vi "Data.Engine.DynamicConfigInitialize.vi"(8 "error in":errorcluster, 10 "Data Access info":T3 {"Read"."Refs"."Data Reference" format="%.0x"; "Write"."Refs"."Data Reference" format="%.0x"; "ReadWrite"."Refs" format="%.0x"}, 11 "Data Access Engine":refnum<class "Data Access Engine.lvclass">) -> (0 "error out":errorcluster, 3 "Data Access Engine":refnum<class "Data Access Engine.lvclass">)   [LabVIEW 2023, in "Data Access Engine.lvlib" / "Data Access Engine.lvclass"]
uses:
  Data Access Engine.lvclass
  Data Access Engine.lvclass/Data Access Engine.ctl
  Access Type Classes/Read/Read.lvclass
  Access Type Classes/Write/Write.lvclass
  Access Type Classes/ReadWrite/ReadWrite.lvclass
  <vilib>/NI VeriStand/Custom Device API/Data Reference.ctl
  <vilib>/NI VeriStand/Custom Device API/Custom Device API.lvlib
  <vilib>/NI VeriStand/Custom Device API/Block Data Reference.ctl
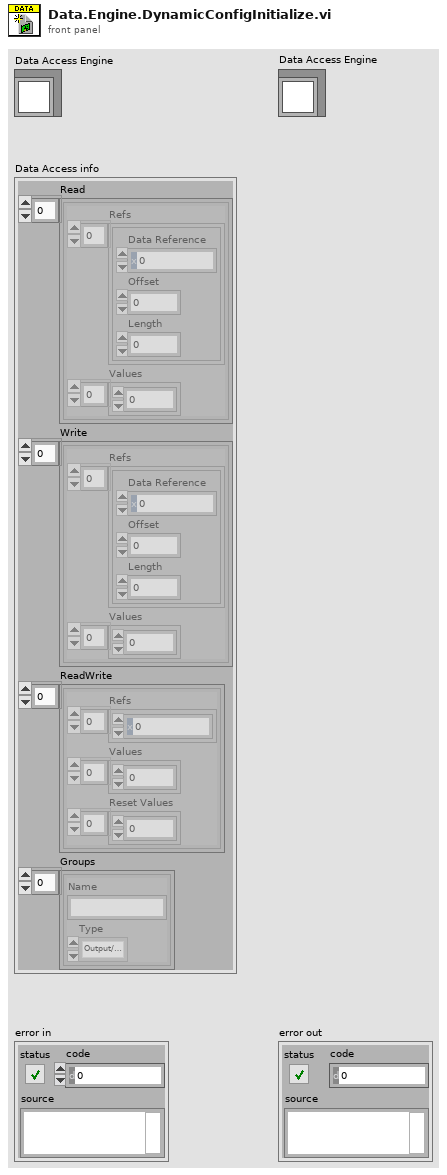
[diagram p1: front panel]
types:
  T1 = typedef "Custom Device API.lvlib/Block Data Reference.ctl" = cluster{"Data Reference":T2, "Offset":u64, "Length":u64}
  T2 = typedef "Custom Device API.lvlib/Data Reference.ctl" = i32
  T3 = cluster{"Read":cluster{"Refs":T1[], "Values":dbl[]}[], "Write":cluster{"Refs":T1[], "Values":dbl[]}[], "ReadWrite":cluster{"Refs":T2[], "Values":dbl[], "Reset Values":dbl[]}[], "Groups":cluster{"Name":string, "Type":enum16{"Output/Write", "Input/Read", "Input/ReadWrite"}}[]}
  T4 = cluster{"Name":string, "Type":enum16{"Output/Write", "Input/Read", "Input/ReadWrite"}}[]
  T5 = cluster{"Refs":T2[], "Values":dbl[], "Reset Values":dbl[]}[]
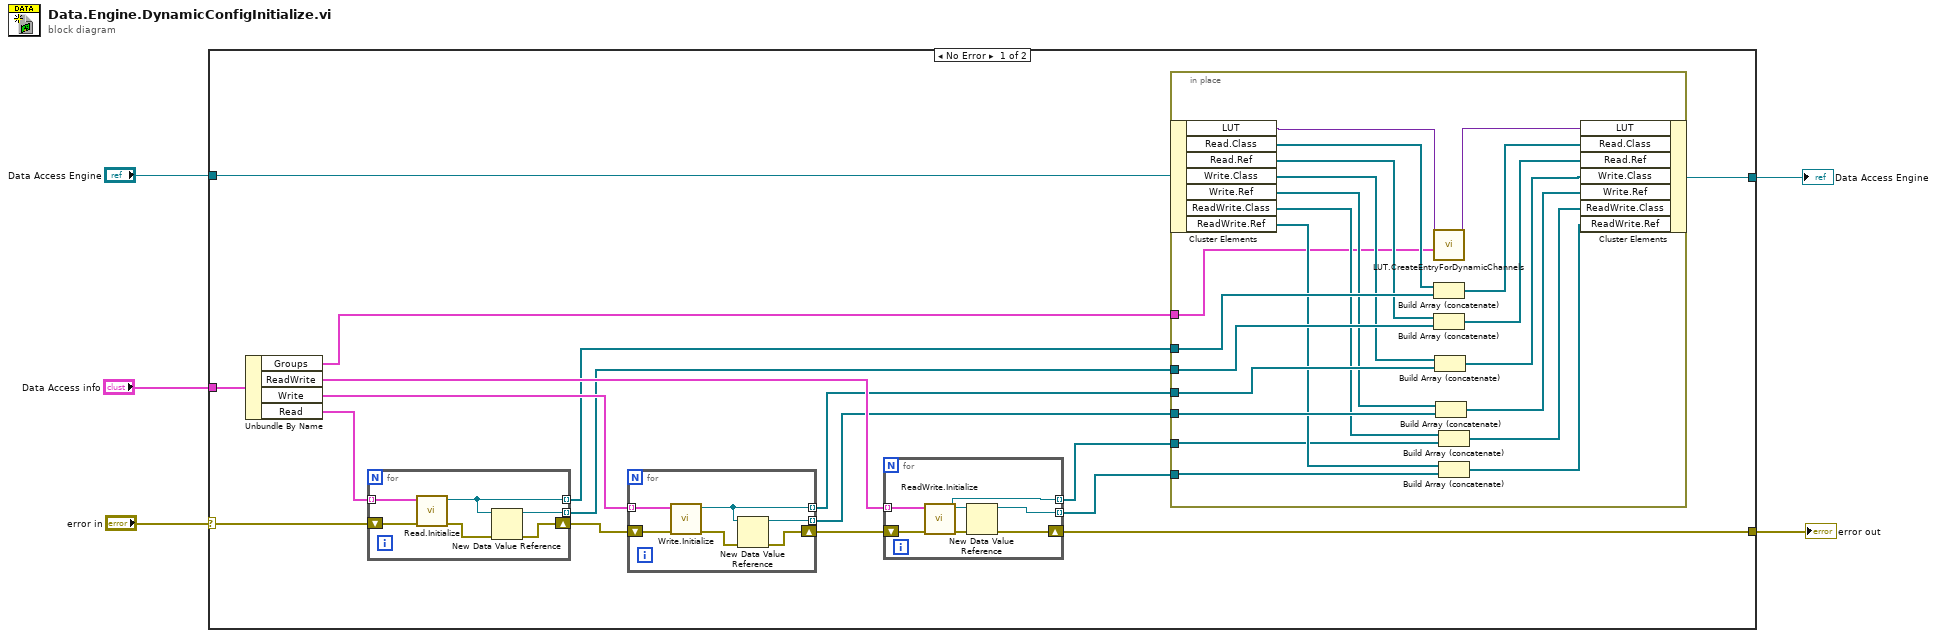
[diagram p0: block diagram]
diagram:
  n1 = case shown="No Error" "error in" {
    selector: "error in" -> [w22 w63]
    tunnel: [w19 w63] -> w4
    tunnel: [w6 w62] -> w3
    tunnel: "Data Access Engine" -> [w8 w62]
    tunnel: "Data Access info" -> [w9 _]
    frame No Error {
      n2 = Unbundle By Name(w9) -> ("Groups"=w7:T4, "ReadWrite"=w16:T5, "Write"=w17:cluster{"Refs":T1[], "Values":dbl[]}[], "Read"=w18:cluster{"Refs":T1[], "Values":dbl[]}[])
      n3 = for {
        tunnel: w18 -> [w29] mode=indexing
        shift-right: [w32] -> w21
        shift-left: w22 -> [w34]
        tunnel: [w31] -> w13 mode=indexing
        tunnel: [w30] -> w10 mode=indexing
        n4 = call "Read.Initialize.vi"("error in (no error)"=w34, "Settings"=w29) -> ("error out"=w33:errorcluster, "Read out"=w31:refnum<class "Read.lvclass">)  [unwired: 8 in]
        n5 = New Data Value Reference(data value=w31, error in=w33) -> (data value reference=w30:refnum<data-value>, error out=w32:errorcluster)
      }
      n6 = for {
        tunnel: w17 -> [w23] mode=indexing
        shift-right: [w26] -> w20
        shift-left: w21 -> [w28]
        tunnel: [w25] -> w14 mode=indexing
        tunnel: [w24] -> w11 mode=indexing
        n7 = call "Write.Initialize.vi"("error in (no error)"=w28, "Settings"=w23) -> ("error out"=w27:errorcluster, "Write out"=w25:refnum<class "Write.lvclass">)  [unwired: 8 in]
        n8 = New Data Value Reference(data value=w25, error in=w27) -> (data value reference=w24:refnum<data-value>, error out=w26:errorcluster)
      }
      n9 = for {
        tunnel: w16 -> [w37] mode=indexing
        shift-right: [w38] -> w19
        shift-left: w20 -> [w40]
        tunnel: [w36] -> w15 mode=indexing
        tunnel: [w35] -> w12 mode=indexing
        n10 = call "ReadWrite.Initialize.vi"("error in (no error)"=w40, "Settings"=w37) -> ("error out"=w39:errorcluster, "ReadWrite out"=w36:refnum<class "ReadWrite.lvclass">)  [unwired: 8 in]
        n11 = New Data Value Reference(data value=w36, error in=w39) -> (data value reference=w35:refnum<data-value>, error out=w38:errorcluster)
      }
      n12 = in-place {
        in-place-border: w15 -> [w52]
        in-place-border: w14 -> [w57]
        in-place-border: w13 -> [w61]
        in-place-border: w12 -> [w51]
        in-place-border: w11 -> [w55]
        in-place-border: w10 -> [w59]
        in-place-border: w7 -> [w41]
        n13 = in-place-cluster #1(w8) -> ("LUT"=w43:variant, "Read.Class"=w50:refnum<class "Read.lvclass">[], "Read.Ref"=w60:refnum<data-value>[], "Write.Class"=w58:refnum<class "Write.lvclass">[], "Write.Ref"=w56:refnum<data-value>[], "ReadWrite.Class"=w54:refnum<class "ReadWrite.lvclass">[], "ReadWrite.Ref"=w53:refnum<data-value>[])
        n14 = call "LUT.CreateEntryForDynamicChannels.vi"("Groups"=w41, "LUT in"=w43) -> ("LUT out"=w42:variant)  [unwired: 8 in, 1 out]
        n15 = Build Array (concatenate)(w50, w61) -> (w49:refnum<class "Read.lvclass">[])
        n16 = Build Array (concatenate)(w60, w59) -> (w48:refnum<data-value>[])
        n17 = Build Array (concatenate)(w58, w57) -> (w47:refnum<class "Write.lvclass">[])
        n18 = Build Array (concatenate)(w56, w55) -> (w46:refnum<data-value>[])
        n19 = Build Array (concatenate)(w54, w52) -> (w45:refnum<class "ReadWrite.lvclass">[])
        n20 = Build Array (concatenate)(w53, w51) -> (w44:refnum<data-value>[])
        n21 = in-place-cluster #1("LUT"=w42, "Read.Class"=w49, "Read.Ref"=w48, "Write.Class"=w47, "Write.Ref"=w46, "ReadWrite.Class"=w45, "ReadWrite.Ref"=w44) -> (w6:refnum<class "Data Access Engine.lvclass">)
      }
    }
    frame Error {
    }
  }
  "error out" <- w4
  "Data Access Engine" <- w3
